vi "Begin.vi"() -> (0 "error out":errorcluster, 1 "CameraDevRef":T1)   [LabVIEW 2011]
doc: "Called before other user functions, this VI is expected to open initial I/O refnums, load in file data, and do all program initialization. Notice that the <B>error out</B> terminal is simply used for data flow. Wiring it to other structures or subVIs ensures that this VI runs first."
uses:
  <vilib>/Rock Robotics/WPI/Camera/WPI_CameraDevRef.ctl
  <vilib>/Rock Robotics/SystemInterfaces/DIO/FPGA_DIOPWMChannel.ctl
  <vilib>/Rock Robotics/WPI/Joystick/WPI_JoystickDeviceEnum.ctl
  <vilib>/Rock Robotics/WPI/Relay/WPI_RelayDirection.ctl
  <vilib>/Rock Robotics/SystemInterfaces/DIO/FPGA_DIORelayChannel.ctl
  <vilib>/Rock Robotics/SystemInterfaces/Typedef/FPGA_TypedefDigitalModule.ctl
  <vilib>/Rock Robotics/SystemInterfaces/AI/FPGA_AIChannel.ctl
  <vilib>/Rock Robotics/SystemInterfaces/AI/FPGA_AIGyroChannel.ctl
  <vilib>/Rock Robotics/SystemInterfaces/DIO/FPGA_DIOChannel.ctl
  <vilib>/Rock Robotics/WPI/Encoder/WPI_EncoderType.ctl
  <vilib>/Rock Robotics/WPI/MotorControl/WPI_MotorControlOpen Jaguar.vi
  <vilib>/Rock Robotics/WPI/MotorControl/WPI_MotorControlOpen Victor.vi
  Robot Global Data.vi
  <vilib>/Rock Robotics/WPI/Counter/WPI_CounterDigitalInputToDigitalSource.vi
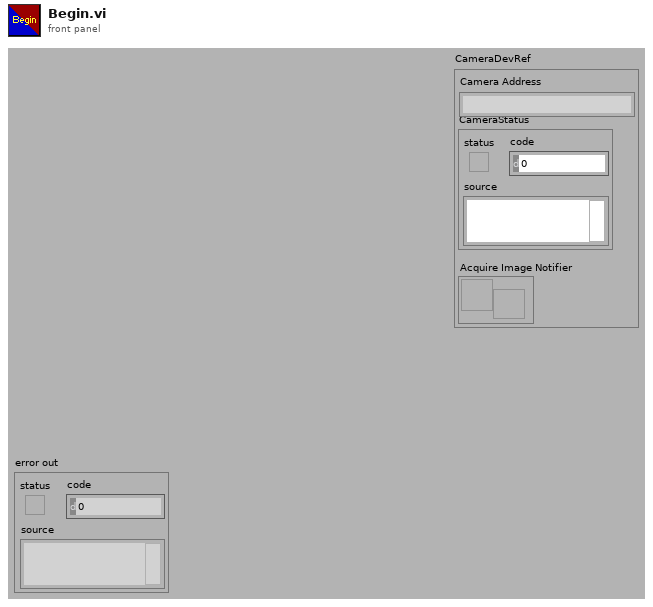
[diagram p1: front panel]
types:
  T1 = typedef "WPI_CameraDevRef.ctl" = cluster{"Camera Address":string, "CameraStatus":errorcluster, "Acquire Image Notifier":refnum<notifier>}
  T2 = typedef "WPI_EncoderType.ctl" = enum16{"1x", "2x", "4x"}
  T3 = typedef "FPGA_DIOChannel.ctl" = enum8{"DIO 1", "DIO 2", "DIO 3", "DIO 4", "DIO 5", "DIO 6", "DIO 7", "DIO 8", "DIO 9", "DIO 10", "DIO 11", "DIO 12", "DIO 13", "DIO 14", "Invalid"}
  T4 = typedef "FPGA_AIGyroChannel.ctl" = enum8{"AI 1", "AI 2", "Invalid"}
  T5 = typedef "FPGA_AIChannel.ctl" = enum8{"AI 1", "AI 2", "AI 3", "AI 4", "AI 5", "AI 6", "AI 7", "AI 8", "Invalid"}
  T6 = typedef "FPGA_TypedefDigitalModule.ctl" = enum16{"Digital Module 1", "Digital Module 2"}
  T7 = typedef "FPGA_DIORelayChannel.ctl" = enum8{"Relay 1", "Relay 2", "Relay 3", "Relay 4", "Relay 5", "Relay 6", "Relay 7", "Relay 8", "Invalid"}
  T8 = typedef "WPI_RelayDirection.ctl" = enum16{"Both directions", "Forward only", "Reverse only"}
  T9 = typedef "WPI_JoystickDeviceEnum.ctl" = enum16{"USB 1", "USB 2", "USB 3", "USB 4", "Kinect 1", "Kinect 2"}
  T10 = typedef "FPGA_DIOPWMChannel.ctl" = enum8{"PWM 1", "PWM 2", "PWM 3", "PWM 4", "PWM 5", "PWM 6", "PWM 7", "PWM 8", "PWM 9", "PWM 10", "Invalid"}
  T11 = typedef "WPI_DigitalInputDevRef.ctl" = cluster{"DevStatus":errorcluster, "DIO Channel":T3, "Digital Module":T6}
  T12 = typedef "FPGA_CounterEncoderSourceConvertionLVSourceType.ctl" = cluster{"DevStatus":errorcluster, "AnalogTriggerMode?":bool, "DigitalMode":cluster{"Digital Module":T6, "DIO Channel":T13}, "AnalogTriggerMode":cluster{"AnalogTriggerIndex":T14, "OutputType":T15}}
  T13 = typedef "FPGA_DIODigitalSourceChannel.ctl" = enum8{"DIO 1", "DIO 2", "DIO 3", "DIO 4", "DIO 5", "DIO 6", "DIO 7", "DIO 8", "DIO 9", "DIO 10", "DIO 11", "DIO 12", "DIO 13", "DIO 14", "Disabled"}
  T14 = typedef "FPGA_AnalogTriggerIndex.ctl" = enum8{"Trig 0", "Trig 1", "Trig 2", "Trig 3", "Trig 4", "Trig 5", "Trig 6", "Trig 7", "Invalid"}
  T15 = typedef "FPGA_AnalogTriggerOutType.ctl" = enum16{"InWindow", "TriggerState", "Rising", "Falling"}
  T16 = typedef "WPI_EncoderDevRef.ctl" = cluster{"DevStatus":errorcluster, "EncoderIndex":T17, "CounterIndex":T18, "DistancePerCount":dbl, "Decoding Type":T2}
  T17 = typedef "FPGA_EncoderIdx.ctl" = enum8{"Enc 0", "Enc 1", "Enc 2", "Enc 3", "Invalid"}
  T18 = typedef "FPGA_CounterCtrSystemIndex.ctl" = enum8{"Ctr 0", "Ctr 1", "Ctr 2", "Ctr 3", "Ctr 4", "Ctr 5", "Ctr 6", "Ctr 7", "Invalid"}
  T19 = typedef "WPI_CameraImageSize.ctl" = enum16{"640x480", "320x240", "160x120"}
  T20 = cluster{"fps":i32, "compression":i32, "Image Size":T19}
  T21 = typedef "WPI_I2CDevRef.ctl" = cluster{"DevStatus":errorcluster, "Digital Module":T6, "Device Address":u8}
  T22 = typedef "WPI_CameraWhite Balance Values.ctl" = enum16{"Auto", "Fixed indoor", "Fixed outdoor 1", "Fixed outdoor 2", "Fixed fluorescent 1", "Fixed fluorescent 2", "Hold current"}
  T23 = typedef "WPI_CameraExposure Values.ctl" = enum16{"Auto", "Flicker-free 50 Hz", "Flicker-free 60 Hz", "Hold current"}
  T24 = typedef "WPI_ServoDeviceRef.ctl" = cluster{"DeviceStatus":errorcluster, "Digital Module":T6, "PWM Channel":T10, "DeadBand":T25}
  T25 = typedef "WPI_PWMDeadband.ctl" = cluster{"Name":string, "maxPositivePwm":i32, "minPositivePwm":i32, "centerPwm":i32, "maxNegativePwm":i32, "minNegativePwm":i32, "angularRange":u16}
  T26 = typedef "WPI_MotorControlDeviceRef.ctl" = cluster{"DeviceStatus":errorcluster, "Type":enum16{"PWM", "CAN"}, "PWM":cluster{"Digital Module":T6, "PWM Channel":T10, "DeadBand":T25}, "CAN":cluster{"Device Number":u8, "Control Mode":T27, "Semaphore":T28, "Max Vout":dbl}, "Invert":bool, "TransformRef":T29, "InvTransformRef":T29}
  T27 = typedef "WPI_CANJaguar_ControlMode.ctl" = enum8{"Percent VBus", "Current", "Speed", "Position", "Voltage"}
  T28 = typedef "Semaphore RefNum" = refnum<k1>
  T29 = typedef "WPI_PWMTransform_ConPane.ctl" = refnum<vi>
  T30 = typedef "WPI_AnalogChannelDevRef.ctl" = cluster{"DevStatus":errorcluster, "Analog Module":T31, "Analog Channel":T5}
  T31 = typedef "FPGA_TypedefAnalogModule.ctl" = enum16{"Analog Module 1", "Analog Module 2"}
  T32 = typedef "WPI_JoystickDevRef.ctl" = cluster{"Device":T9}
  T33 = typedef "WPI_GyroDevRef.ctl" = cluster{"DevStatus":errorcluster, "Analog Module":T31, "Analog Channel":T5, "Offset":dbl, "Gain (VoltsPerDegree/Second)":dbl}
  T34 = typedef "WPI_RelayDevRef.ctl" = cluster{"DevStatus":errorcluster, "Relay Channel":T7, "Digital Module":T6, "Relay Direction":T8}
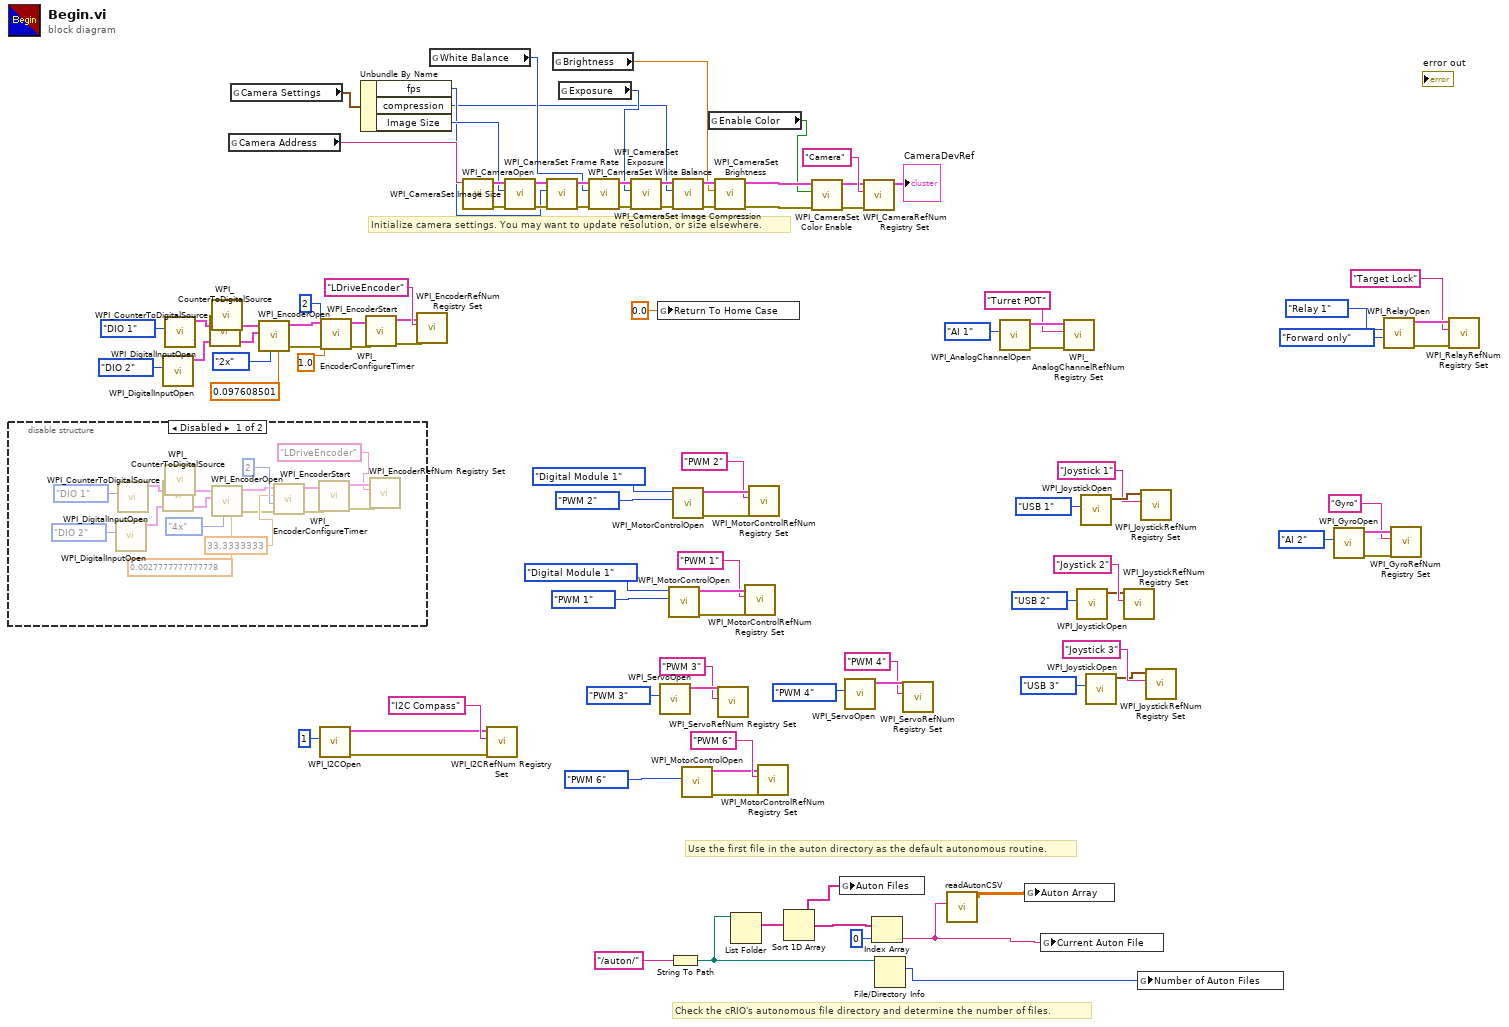
[diagram p0: block diagram]
diagram:
  # "Check the cRIO's autonomous file directory and determine the number of files."
  # "Use the first file in the auton directory as the default autonomous routine."
  # "Initialize camera settings. You may want to update resolution, or size elsewhere."
  n1 = disable-structure shown="Disabled" {
    frame Disabled {
      n2 = call <vilib>:"WPI_DigitalInputOpen.vi"("DIO Channel"=FPGA_DIOChannel."DIO 2") -> ("DigitalInputDevRef"=w105:T11)  [unwired: 9 in, 1 out]
      n3 = call <vilib>:"WPI_DigitalInputOpen.vi"("DIO Channel"=FPGA_DIOChannel."DIO 1") -> ("DigitalInputDevRef"=w102:T11)  [unwired: 9 in, 1 out]
      n4 = call-poly <vilib>:"WPI_CounterToDigitalSource.vi"("DigitalInputDevRef"=w105) -> ("Digital Source"=w106:T12)  [unwired: 6 in]
      n5 = call-poly <vilib>:"WPI_CounterToDigitalSource.vi"("DigitalInputDevRef"=w102) -> ("Digital Source"=w101:T12)  [unwired: 6 in]
      n6 = call <vilib>:"WPI_EncoderOpen.vi"("DistancePerCount"=0.0027777777777778, "Decoding Type"=WPI_EncoderType."4x", "BSource"=w106, "ASource"=w101) -> ("error out"=w109:errorcluster, "EncoderDevRef"=w110:T16)  [unwired: 6 in]
      n7 = call <vilib>:"WPI_EncoderConfigureTimer.vi"("error in (no error)"=w109, "Number Samples to Average"=u8 2, "Minimum Rate"=33.3333333, "EncoderDevRef"=w110) -> ("error out"=w114:errorcluster, "EncoderDevRef"=w113:T16)  [unwired: 6 in]
      n8 = call <vilib>:"WPI_EncoderStart.vi"("error in (no error)"=w114, "EncoderDevRef"=w113) -> ("error out"=w116:errorcluster, "EncoderDevRef"=w115:T16)  [unwired: 8 in]
      n9 = call <vilib>:"WPI_EncoderRefNum Registry Set.vi"("error in (no error)"=w116, "refnum name"="LDriveEncoder", "EncoderDevRef"=w115) -> ()  [unwired: 7 in, 2 out]
    }
    frame Enabled {
    }
  }
  n10 = call <vilib>:"WPI_DigitalInputOpen.vi"("DIO Channel"=FPGA_DIOChannel."DIO 2") -> ("DigitalInputDevRef"=w13:T11)  [unwired: 9 in, 1 out]
  n11 = call <vilib>:"WPI_DigitalInputOpen.vi"("DIO Channel"=FPGA_DIOChannel."DIO 1") -> ("DigitalInputDevRef"=w16:T11)  [unwired: 9 in, 1 out]
  n12 = call-poly <vilib>:"WPI_CounterToDigitalSource.vi"("DigitalInputDevRef"=w13) -> ("Digital Source"=w12:T12)  [unwired: 6 in]
  n13 = call-poly <vilib>:"WPI_CounterToDigitalSource.vi"("DigitalInputDevRef"=w16) -> ("Digital Source"=w17:T12)  [unwired: 6 in]
  n14 = global read "Robot Global Data.vi" "Camera Address"() -> (w86:string)
  n15 = global read "Robot Global Data.vi" "Camera Settings"() -> (w58:T20)
  n16 = call <vilib>:"WPI_EncoderOpen.vi"("DistancePerCount"=0.097608501, "Decoding Type"=WPI_EncoderType."2x", "BSource"=w12, "ASource"=w17) -> ("error out"=w8:errorcluster, "EncoderDevRef"=w7:T16)  [unwired: 6 in]
  n17 = call <vilib>:"WPI_I2COpen.vi"("Device Address"=u8 1) -> ("error out"=w18:errorcluster, "I2CDevRef"=w19:T21)  [unwired: 9 in]
  n18 = call <vilib>:"WPI_EncoderConfigureTimer.vi"("error in (no error)"=w8, "Number Samples to Average"=u8 2, "Minimum Rate"=1.0, "EncoderDevRef"=w7) -> ("error out"=w3:errorcluster, "EncoderDevRef"=w4:T16)  [unwired: 6 in]
  n19 = Unbundle By Name(w58) -> ("fps"=w56:i32, "compression"=w53:i32, "Image Size"=w57:T19)
  n20 = call <vilib>:"WPI_EncoderStart.vi"("error in (no error)"=w3, "EncoderDevRef"=w4) -> ("error out"=w1:errorcluster, "EncoderDevRef"=w2:T16)  [unwired: 8 in]
  n21 = call <vilib>:"WPI_EncoderRefNum Registry Set.vi"("error in (no error)"=w1, "refnum name"="LDriveEncoder", "EncoderDevRef"=w2) -> ()  [unwired: 7 in, 2 out]
  n22 = global read "Robot Global Data.vi" "White Balance"() -> (w55:T22)
  n23 = call <vilib>:"WPI_CameraOpen.vi"("Camera Address"=w86) -> ("error out"=w92:errorcluster, "CameraDevRef"=w93:T1)  [unwired: 1 in, 8 out]
  n24 = call <vilib>:"WPI_I2CRefNum Registry Set.vi"("error in (no error)"=w18, "refnum name"="I2C Compass", "I2CDevRef"=w19) -> ()  [unwired: 7 in, 2 out]
  n25 = call <vilib>:"WPI_CameraSet Image Size.vi"("error in (no error)"=w92, "Image Size"=w57, "CameraDevRef"=w93) -> ("error out"=w91:errorcluster, "CameraDevRef Out"=w94:T1)  [unwired: 7 out]
  n26 = call <vilib>:"WPI_CameraSet Frame Rate.vi"("error in (no error)"=w91, "Frame Rate (fps)"=w56, "CameraDevRef"=w94) -> ("error out"=w90:errorcluster, "CameraDevRef Out"=w96:T1)  [unwired: 7 out]
  n27 = global read "Robot Global Data.vi" "Brightness"() -> (w52:dbl)
  n28 = global read "Robot Global Data.vi" "Exposure"() -> (w54:T23)
  n29 = call <vilib>:"WPI_CameraSet White Balance.vi"("error in (no error)"=w90, "White Balance"=w55, "CameraDevRef"=w96) -> ("error out"=w89:errorcluster, "CameraDevRef Out"=w95:T1)  [unwired: 7 out]
  n30 = call <vilib>:"WPI_CameraSet Exposure.vi"("error in (no error)"=w89, "Exposure"=w54, "CameraDevRef"=w95) -> ("error out"=w88:errorcluster, "CameraDevRef Out"=w98:T1)  [unwired: 7 out]
  n31 = global write "Robot Global Data.vi" "Return To Home Case"(0.0 ("Return To Home Case")) -> ()
  n32 = call <vilib>:"WPI_ServoOpen.vi"("PWM Channel"=FPGA_DIOPWMChannel."PWM 3") -> ("ServoDeviceRef"=w72:T24)  [unwired: 9 in, 1 out]
  n33 = call-poly <vilib>:"WPI_MotorControlOpen.vi"("PWM Channel"=FPGA_DIOPWMChannel."PWM 1", "Digital Module (Module 1)"=FPGA_TypedefDigitalModule."Digital Module 1") -> ("error out"=w78:errorcluster, "MotorControlDeviceRef"=w81:T26)  [unwired: 8 in]
  n34 = String To Path(string="/auton/") -> (path=w32:path)
  n35 = call <vilib>:"WPI_CameraSet Image Compression.vi"("error in (no error)"=w88, "Compression"=w53, "CameraDevRef"=w98) -> ("error out"=w87:errorcluster, "CameraDevRef Out"=w97:T1)  [unwired: 7 out]
  n36 = call-poly <vilib>:"WPI_MotorControlOpen.vi"("PWM Channel"=FPGA_DIOPWMChannel."PWM 2", "Digital Module (Module 1)"=FPGA_TypedefDigitalModule."Digital Module 1") -> ("error out"=w79:errorcluster, "MotorControlDeviceRef"=w84:T26)  [unwired: 8 in]
  n37 = call-poly <vilib>:"WPI_MotorControlOpen.vi"("PWM Channel"=FPGA_DIOPWMChannel."PWM 6") -> ("error out"=w67:errorcluster, "MotorControlDeviceRef"=w65:T26)  [unwired: 9 in]
  n38 = global read "Robot Global Data.vi" "Enable Color"() -> (w47:bool)
  n39 = call <vilib>:"WPI_CameraSet Brightness.vi"("error in (no error)"=w87, "Brightness"=w52, "CameraDevRef"=w97) -> ("error out"=w50:errorcluster, "CameraDevRef Out"=w51:T1)  [unwired: 7 out]
  n40 = call <vilib>:"WPI_ServoRefNum Registry Set.vi"("refnum name"="PWM 3", "ServoDeviceRef"=w72) -> ()  [unwired: 8 in, 2 out]
  n41 = List Folder(path=w32) -> (filenames=w31:string[])  [unwired: 1 in, 5 out]
  n42 = call <vilib>:"WPI_MotorControlRefNum Registry Set.vi"("error in (no error)"=w78, "refnum name"="PWM 1", "MotorControlDevRef"=w81) -> ()  [unwired: 7 in, 2 out]
  n43 = call <vilib>:"WPI_MotorControlRefNum Registry Set.vi"("error in (no error)"=w79, "refnum name"="PWM 2", "MotorControlDevRef"=w84) -> ()  [unwired: 7 in, 2 out]
  n44 = call <vilib>:"WPI_MotorControlRefNum Registry Set.vi"("error in (no error)"=w67, "refnum name"="PWM 6", "MotorControlDevRef"=w65) -> ()  [unwired: 7 in, 2 out]
  n45 = Sort 1D Array(array=w31) -> (sorted array=w26:string[])
  n46 = call <vilib>:"WPI_CameraSet Color Enable.vi"("error in (no error)"=w50, "Color Enabled"=w47, "CameraDevRef"=w51) -> ("error out"=w48:errorcluster, "CameraDevRef Out"=w49:T1)  [unwired: 7 in]
  n47 = global write "Robot Global Data.vi" "Auton Files"(w26) -> ()
  n48 = call <vilib>:"WPI_ServoOpen.vi"("PWM Channel"=FPGA_DIOPWMChannel."PWM 4") -> ("ServoDeviceRef"=w70:T24)  [unwired: 9 in, 1 out]
  n49 = call <vilib>:"WPI_CameraRefNum Registry Set.vi"("error in (no error)"=w48, "refnum name"="Camera", "CameraDevRef"=w49) -> ("CameraDevRef"=→"CameraDevRef":T1)  [unwired: 8 out]
  n50 = Index Array(array=w26, index=0) -> (element=w28:string)
  n51 = File/Directory Info(path=w32) -> (size=w29:i64)  [unwired: 1 in, 6 out]
  n52 = call <vilib>:"WPI_ServoRefNum Registry Set.vi"("refnum name"="PWM 4", "ServoDeviceRef"=w70) -> ()  [unwired: 8 in, 2 out]
  n53 = call "readAutonCSV.vi"("AutonFile"=w28) -> ("AutonArray"=w27:dbl[][])  [unwired: 7 in]
  n54 = call <vilib>:"WPI_AnalogChannelOpen.vi"("Analog Channel"=FPGA_AIChannel."AI 1") -> ("error out"=w37:errorcluster, "AIDeviceRef"=w38:T30)  [unwired: 9 in]
  n55 = global write "Robot Global Data.vi" "Auton Array"(w27) -> ()
  n56 = global write "Robot Global Data.vi" "Current Auton File"(w28) -> ()
  n57 = call <vilib>:"WPI_AnalogChannelRefNum Registry Set.vi"("error in (no error)"=w37, "refnum name"="Turret POT", "AIDeviceRef"=w38) -> ()  [unwired: 7 in, 2 out]
  n58 = call <vilib>:"WPI_JoystickOpen.vi"("JoystickDevice"=WPI_JoystickDeviceEnum."USB 2") -> ("JoystickDevRef"=w74:T32)  [unwired: 10 in]
  n59 = call <vilib>:"WPI_JoystickOpen.vi"("JoystickDevice"=WPI_JoystickDeviceEnum."USB 1") -> ("JoystickDevRef"=w77:T32)  [unwired: 10 in]
  n60 = call <vilib>:"WPI_JoystickOpen.vi"("JoystickDevice"=WPI_JoystickDeviceEnum."USB 3") -> ("JoystickDevRef"=w62:T32)  [unwired: 10 in]
  n61 = call <vilib>:"WPI_JoystickRefNum Registry Set.vi"("refnum name"="Joystick 2", "JoystickDevRef"=w74) -> ()  [unwired: 8 in, 2 out]
  n62 = global write "Robot Global Data.vi" "Number of Auton Files"(w29) -> ()
  n63 = call <vilib>:"WPI_JoystickRefNum Registry Set.vi"("refnum name"="Joystick 1", "JoystickDevRef"=w77) -> ()  [unwired: 8 in, 2 out]
  n64 = call <vilib>:"WPI_JoystickRefNum Registry Set.vi"("refnum name"="Joystick 3", "JoystickDevRef"=w62) -> ()  [unwired: 8 in, 2 out]
  n65 = call <vilib>:"WPI_GyroOpen.vi"("Analog Channel"=FPGA_AIGyroChannel."AI 2") -> ("error out"=w25:errorcluster, "GyroDevRef"=w24:T33)  [unwired: 8 in, 1 out]
  n66 = call <vilib>:"WPI_RelayOpen.vi"("Relay Direction"=WPI_RelayDirection."Forward only", "Relay Channel"=FPGA_DIORelayChannel."Relay 1") -> ("error out"=w44:errorcluster, "RelayDevRef"=w45:T34)  [unwired: 8 in]
  n67 = call <vilib>:"WPI_GyroRefNum Registry Set.vi"("error in (no error)"=w25, "refnum name"="Gyro", "GyroDevRef"=w24) -> ()  [unwired: 7 in, 2 out]
  n68 = call <vilib>:"WPI_RelayRefNum Registry Set.vi"("error in (no error)"=w44, "refnum name"="Target Lock", "RelayDevRef"=w45) -> ()  [unwired: 7 in, 2 out]
